vi "Test Result.vi"(8 "error in":errorcluster, 10 "Test Result payload":T1, 11 "Module ID":i32=-1) -> (0 "error out":errorcluster)   [LabVIEW 2021, in "MQTT Bridge.lvlib"]
doc: "_____\nCreated using DQMH Framework: Event Scripter 7.1.1.1528."
uses:
  MQTT Bridge.lvlib
  Test Result Payload.ctl
  Test Result Argument--cluster.ctl
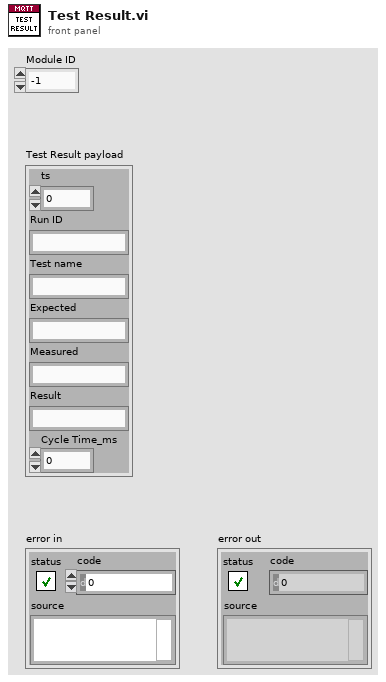
[diagram p1: front panel]
types:
  T1 = typedef "Test Result Payload.ctl" = cluster{"ts":dbl, "Run ID":string, "Test name":string, "Expected":string, "Measured":string, "Result":string, "Cycle Time_ms":u16}
  T2 = typedef "MQTT Bridge.lvlib/Test Result Argument--cluster.ctl" = cluster{"Module ID":i32, "Test Result payload":T1}
  T3 = typedef "MQTT Bridge.lvlib/Request Events--cluster.ctl" = cluster{"Stop Module":refnum<user-event>, "Show Panel":refnum<user-event>, "Hide Panel":refnum<user-event>, "Show Diagram":refnum<user-event>, "Get Module Execution Status":refnum<user-event>, "Connect":refnum<user-event>, "Subscribe":refnum<user-event>, "Update Client Data":refnum<user-event>, "Disconnect":refnum<user-event>, "Check Connection":refnum<user-event>, "Ack Variable Write":refnum<user-event>, "Ack Run Start":refnum<user-event>, "Get Recipe":refnum<user-event>, "Run Finished":refnum<user-event>, "Test Result":refnum<user-event>}
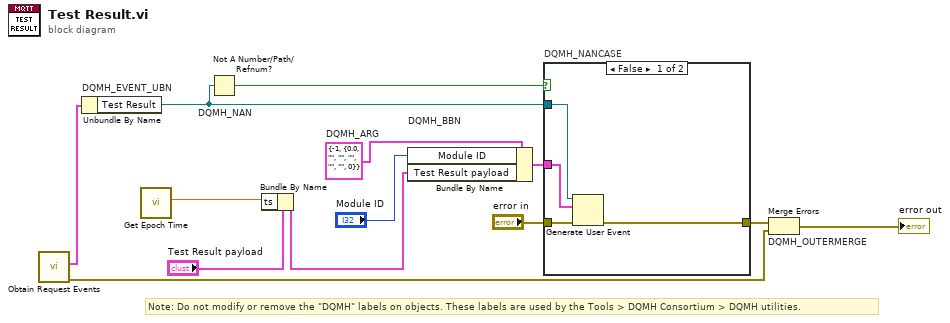
[diagram p0: block diagram]
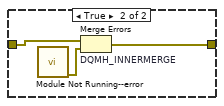
[diagram p2: hidden frame]
diagram:
  w7 = T2 {"Module ID"=-1, "Test Result payload"={"ts"=0.0, "Run ID"="", "Test name"="", "Expected"="", "Measured"="", "Result"="", "Cycle Time_ms"=0}}  # DQMH_ARG
  # "Note: Do not modify or remove the \"DQMH\" labels on objects. These labels are used by the Tools > DQMH Consortium > DQMH utilities."
  n1 = call "Obtain Request Events.vi"() -> ("error out"=w4:errorcluster, "MQTT Bridge Request Events"=w3:T3)  [unwired: 10 in]
  n2 = Unbundle By Name "DQMH_EVENT_UBN"(w3) -> ("Test Result"=w9:refnum<user-event>)
  n3 = call "Get Epoch Time.vi"() -> ("double precision float"=w1:dbl)  [unwired: 11 in]
  n4 = Not A Number/Path/Refnum? "DQMH_NAN"(number/path/refnum=w9) -> (NaN/Path/Refnum?=w10:bool)
  n5 = Bundle By Name(cluster="Test Result payload", "ts"=w1) -> (w2:T1)
  n6 = Bundle By Name "DQMH_BBN"(cluster=w7, "Module ID"="Module ID", "Test Result payload"=w2) -> (w11:T2)
  n7 = case "DQMH_NANCASE" shown="False" w10 {
    tunnel: "error in" -> [w17 w20]
    tunnel: [w16 w19] -> w8
    tunnel: w9 -> [w15 _]
    tunnel: w11 -> [w14 _]
    frame False {
      n8 = Generate User Event(user event=w15, event data cluster=w14, error in=w17) -> (error out=w16:errorcluster)  [unwired: 1 in, 1 out]
    }
    frame True {
      n9 = call "Module Not Running--error.vi"() -> ("error out"=w18:errorcluster)  [unwired: 11 in]
      n10 = Merge Errors "DQMH_INNERMERGE"(w20, w18) -> (w19:errorcluster)
    }
  }
  n11 = Merge Errors "DQMH_OUTERMERGE"(w8, w4) -> (→"error out":errorcluster)
